vi "_PC_Daemon_Turbo stateMachine.vi"(5 "state":T1, 7 "engMode":bool, 8 "error in":errorcluster, 10 "newData":variant, 11 "refnumCluster":T2) -> (0 "error out":errorcluster)   [LabVIEW 2018]
uses:
  turboState.ctl
  RT/PublicSubVI/Ctl/_ctl_RT_TurboSettings.ctl
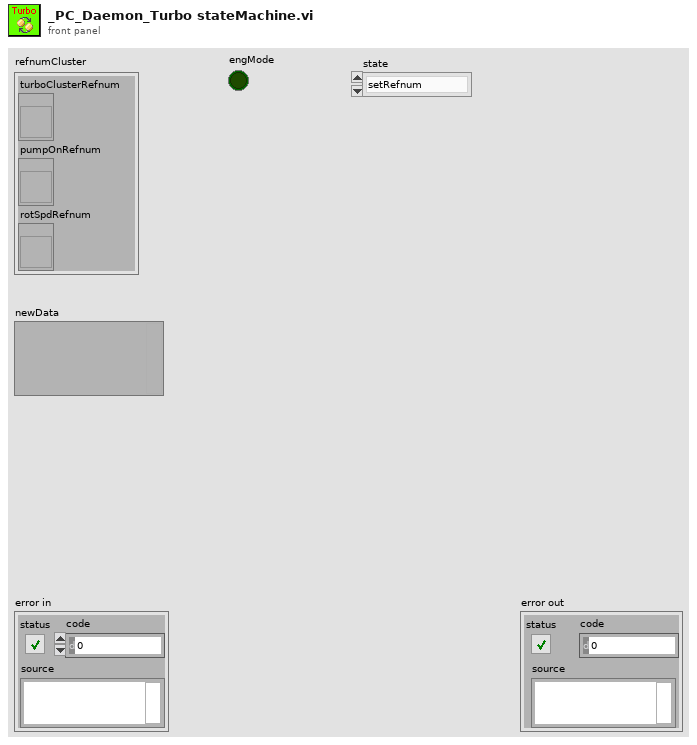
[diagram p1: front panel]
types:
  T1 = typedef "turboState.ctl" = enum16{"setRefnum", "init", "setParam", "close"}
  T2 = cluster{"turboClusterRefnum":refnum<vi>, "pumpOnRefnum":refnum<vi>, "rotSpdRefnum":refnum<vi>}
  T3 = typedef "_ctl_RT_TurboSettings.ctl" = cluster{"Preset rot. speed \nat standby mode(%)":dbl, "Speed set value in rot. speed \nsetting operations (%)":dbl, "Max. power (%)":dbl, "Gas mode: ":enum16{"heavy", "light", "helium"}, "Operations mode: ":bool, "Motor turbopump: ":bool, "Pumping station: ":bool, "Standby: ":bool, "Timestamp":timestamp}
  T4 = cluster{"Preset rot. speed \nat standby mode(%)":dbl, "Speed set value in rot. speed \nsetting operations (%)":dbl, "Max. power (%)":dbl, "Gas mode: ":enum16{"heavy", "light", "helium"}, "Operations mode: ":bool, "Motor turbopump: ":bool, "Pumping station: ":bool, "Standby: ":bool}
  T5 = enum8{"Enabled", "Disabled", "Disabled and Grayed Out"}
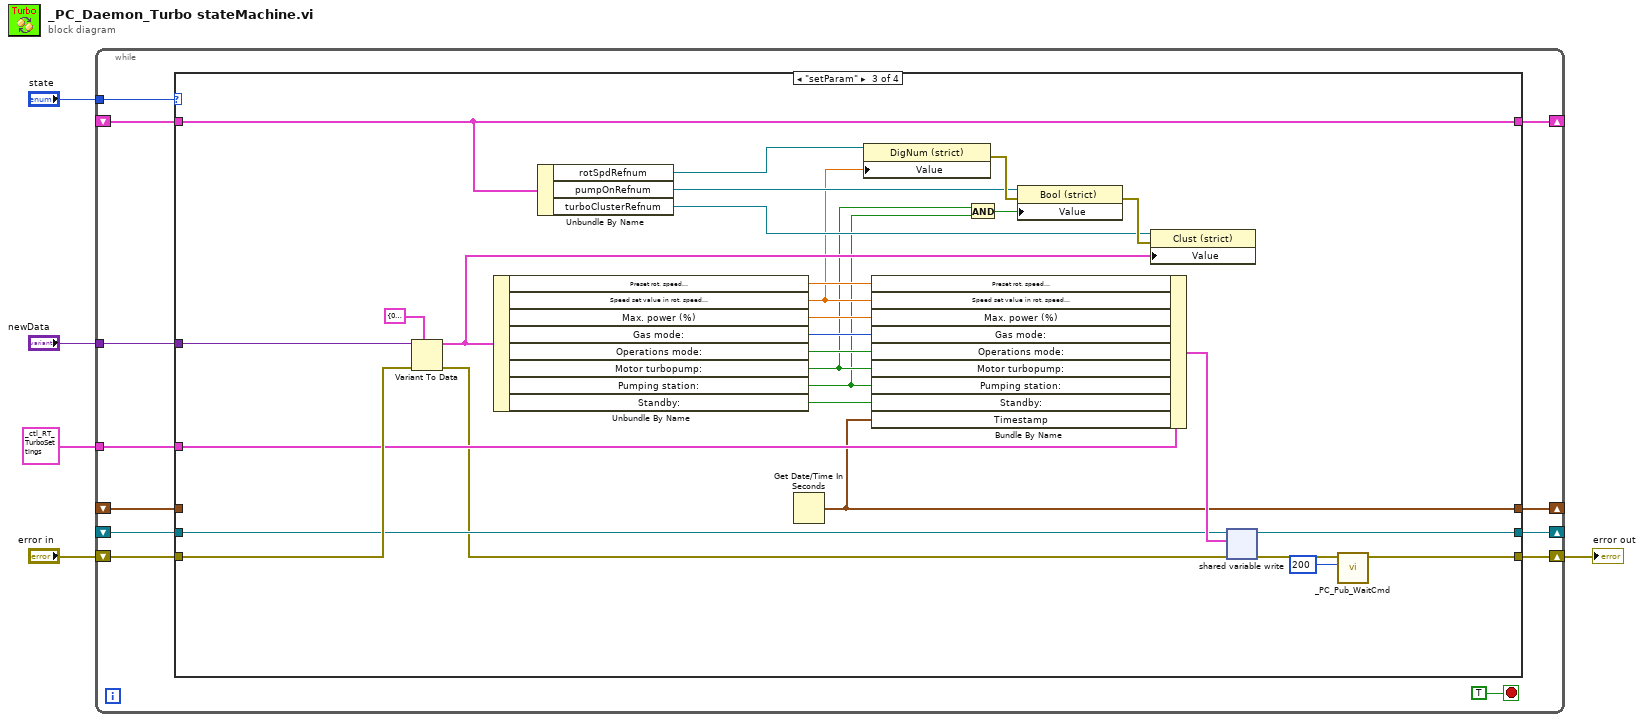
[diagram p0: block diagram]
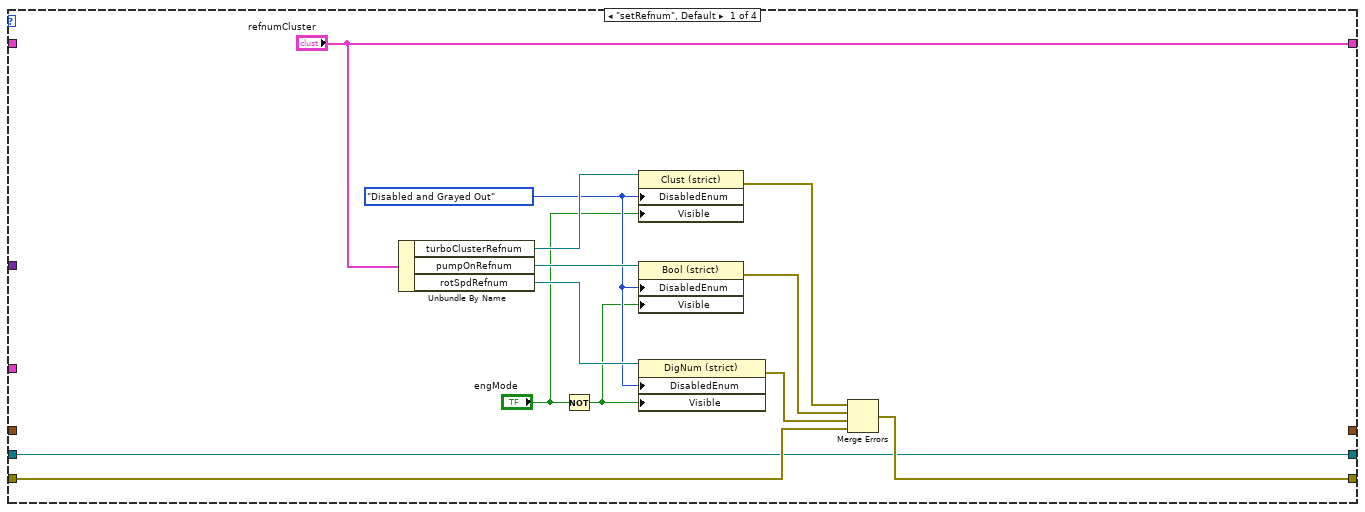
[diagram p2: hidden frame]
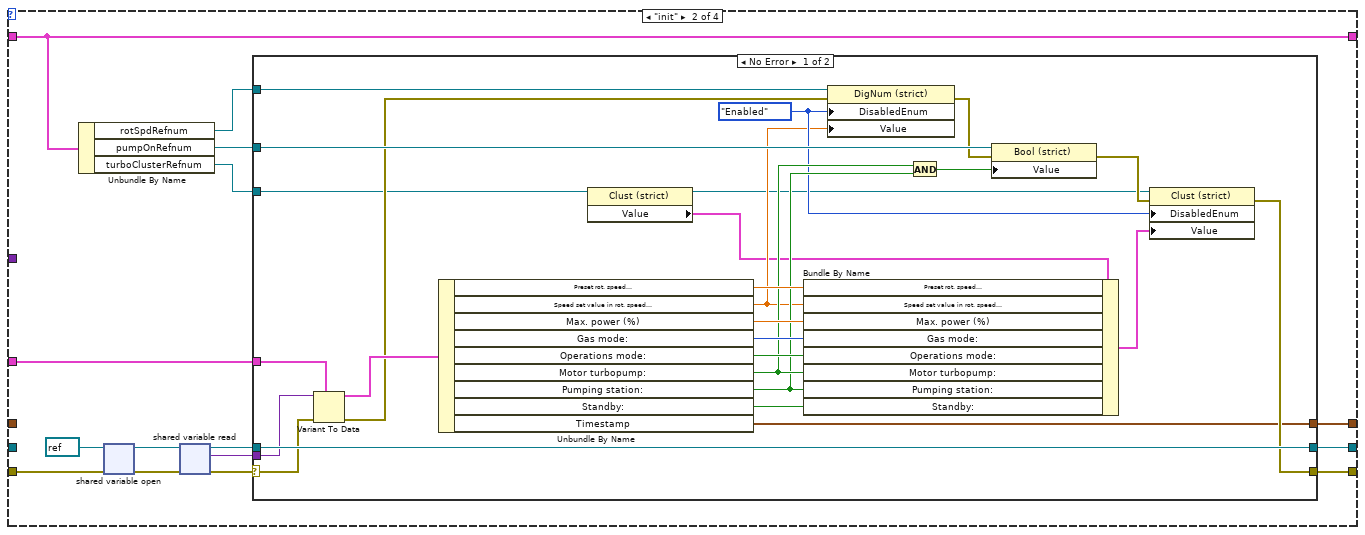
[diagram p3: hidden frame]
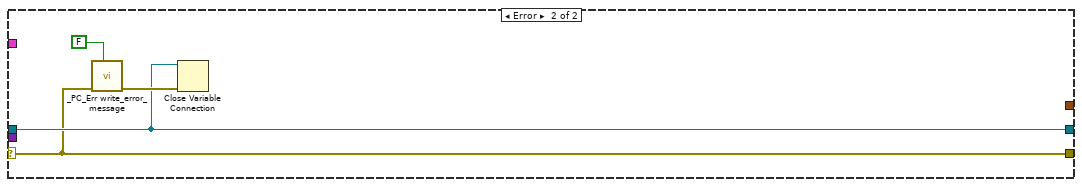
[diagram p4: hidden frame]
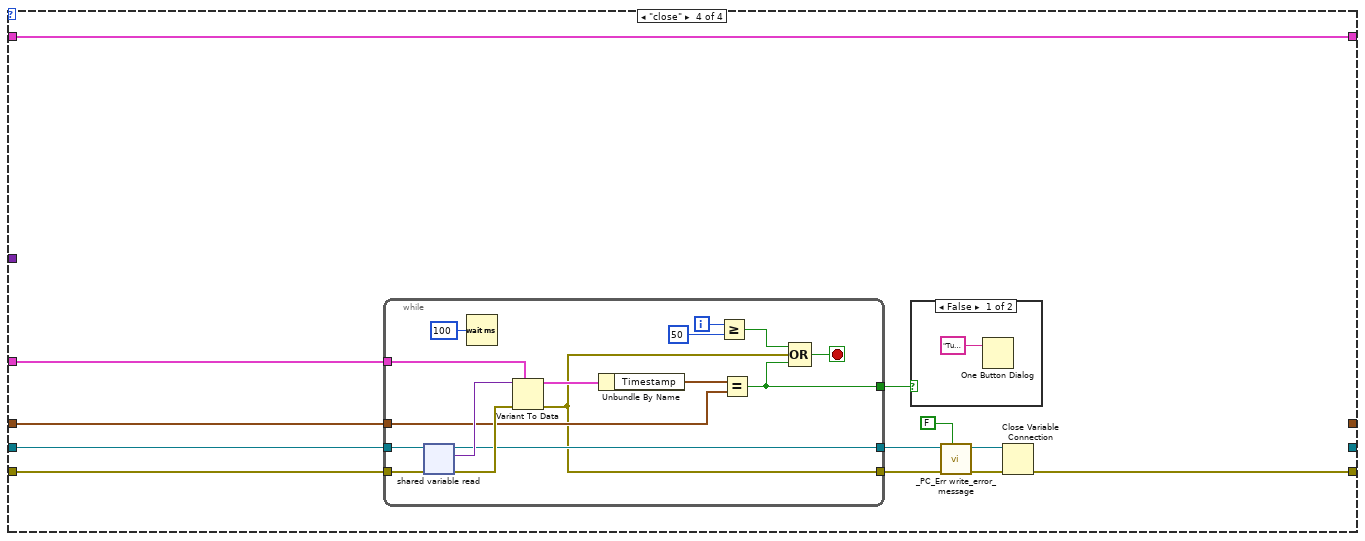
[diagram p5: hidden frame]
diagram:
  n1 = while {
    tunnel: "state" -> [w17]
    shift-right: [w16] -> _
    shift-left: _ -> [w13]
    shift-right: [w15] -> w2
    shift-left: "error in" -> [w14]
    tunnel: T3 {"Preset rot. speed \nat standby mode(%)"=0.0, "Speed set value in rot. speed \nsetting operations (%)"=0.0, "Max. power (%)"=0.0, "Gas mode: "=enum."heavy", "Operations mode: "=FALSE, "Motor turbopump: "=FALSE, "Pumping station: "=FALSE, "Standby: "=FALSE, "Timestamp"=timestamp(0 s since 1904-01-01)} ("TurboSettings") -> [w12]
    shift-right: [w11] -> _
    shift-left: _ -> [w10]
    tunnel: "newData" -> [w9]
    shift-right: [w7] -> _
    shift-left: _ -> [w6]
    stop <- TRUE stop-if-true
    n2 = case shown="\"setParam\"" w17 {
      tunnel: ["refnumCluster" w36 w87 w111] -> w16
      tunnel: [w20 w35 w77 w105] -> w15
      tunnel: w14 -> [w19 w32 w101 w113]
      tunnel: w13 -> [_ w36 w87 w111]
      tunnel: w12 -> [_ w40 w100 w110]
      tunnel: [w18 w34 w80 _] -> w11
      tunnel: w10 -> [w18 _ w82 w114]
      tunnel: w9 -> [_ _ w102 _]
      tunnel: [_ w31 w76 _] -> w7
      tunnel: w6 -> [_ _ _ w112]
      frame "setRefnum", Default {
        w26 = T5."Disabled and Grayed Out" ("Disabled")
        n3 = Unbundle By Name("refnumCluster") -> ("turboClusterRefnum"=w27:refnum<vi>, "pumpOnRefnum"=w28:refnum<vi>, "rotSpdRefnum"=w29:refnum<vi>)
        n4 = Not(x="engMode") -> (.not. x?=w25:bool)
        n5 = property class="Clust (strict)"(reference=w27, "DisabledEnum"=w26, "Visible"="engMode") -> (error out=w23:errorcluster)  [unwired: 1 in, 1 out]
        n6 = property class="Bool (strict)"(reference=w28, "DisabledEnum"=w26, "Visible"=w25) -> (error out=w22:errorcluster)  [unwired: 1 in, 1 out]
        n7 = property class="DigNum (strict)"(reference=w29, "DisabledEnum"=w26, "Visible"=w25) -> (error out=w21:errorcluster)  [unwired: 1 in, 1 out]
        n8 = Merge Errors(w23, w22, w21, w19) -> (w20:errorcluster)
      }
      frame "init" {
        n9 = Unbundle By Name(w36) -> ("rotSpdRefnum"=w37:refnum<vi>, "pumpOnRefnum"=w38:refnum<vi>, "turboClusterRefnum"=w39:refnum<vi>)
        n10 = shared-variable-open(refnum<k21> "ni.var.psp://NI-sbRIO/_RT_CtrlLoop_TurboPump_Variables/TurboSettings" ("shared variable refnum in"), w32) -> (w45:refnum<k21>, w44:errorcluster)
        n11 = shared-variable-read(w45, w44) -> (w43:refnum<k21>, w41:errorcluster, w42:variant)
        n12 = case shown="No Error" w41 {
          selector: w41 -> [w69 w72]
          tunnel: w43 -> [w71 w73]
          tunnel: [w71 w73] -> w34
          tunnel: w42 -> [w70 _]
          tunnel: w39 -> [w51 _]
          tunnel: w38 -> [w61 _]
          tunnel: w37 -> [w57 _]
          tunnel: w40 -> [w48 _]
          tunnel: [w47 w72] -> w35
          tunnel: [w46 _] -> w31
          frame No Error {
            w56 = T5."Enabled" ("Disabled")
            n13 = Variant To Data(error in=w69, type=w48, Variant=w70) -> (data=w68:T3, error out=w54:errorcluster)
            n14 = Unbundle By Name(w68) -> ("Preset rot. speed \nat standby mode(%)"=w67:dbl, "Speed set value in rot. speed \nsetting operations (%)"=w55:dbl, "Max. power (%)"=w66:dbl, "Gas mode:"=w65:enum16{"heavy", "light", "helium"}, "Operations mode:"=w64:bool, "Motor turbopump:"=w60:bool, "Pumping station:"=w59:bool, "Standby:"=w63:bool, "Timestamp"=w46:timestamp)
            n15 = property class="Clust (strict)"(reference=w51) -> (reference out=w50:refnum<vi>, "Value"=w49:T4)  [unwired: 1 in, 1 out]
            n16 = Bundle By Name(cluster=w49, "Preset rot. speed \nat standby mode(%)"=w67, "Speed set value in rot. speed \nsetting operations (%)"=w55, "Max. power (%)"=w66, "Gas mode:"=w65, "Operations mode:"=w64, "Motor turbopump:"=w60, "Pumping station:"=w59, "Standby:"=w63) -> (w62:T4)
            n17 = property class="DigNum (strict)"(reference=w57, error in=w54, "DisabledEnum"=w56, "Value"=w55) -> (error out=w53:errorcluster)  [unwired: 1 out]
            n18 = And(x=w60, y=w59) -> (x .and. y?=w58:bool)
            n19 = property class="Bool (strict)"(reference=w61, error in=w53, "Value"=w58) -> (error out=w52:errorcluster)  [unwired: 1 out]
            n20 = property class="Clust (strict)"(reference=w50, error in=w52, "DisabledEnum"=w56, "Value"=w62) -> (error out=w47:errorcluster)  [unwired: 1 out]
          }
          frame Error {
            n21 = call "_PC_Err write_error_message.vi"("show msg( T )"=FALSE, "error in"=w72) -> ("error out"=w75:errorcluster)  [unwired: 9 in]
            n22 = Close Variable Connection(8:w75, 11:w73) -> ()  [unwired: 1 out]
          }
        }
      }
      frame "setParam" {
        n23 = Variant To Data(error in=w101, type=T4 {"Preset rot. speed \nat standby mode(%)"=0.0, "Speed set value in rot. speed \nsetting operations (%)"=0.0, "Max. power (%)"=0.0, "Gas mode: "=enum."heavy", "Operations mode: "=FALSE, "Motor turbopump: "=FALSE, "Pumping station: "=FALSE, "Standby: "=FALSE} ("TC110 Settings"), Variant=w102) -> (data=w88:T4, error out=w81:errorcluster)
        n24 = Unbundle By Name(w88) -> ("Preset rot. speed \nat standby mode(%)"=w99:dbl, "Speed set value in rot. speed \nsetting operations (%)"=w86:dbl, "Max. power (%)"=w98:dbl, "Gas mode:"=w97:enum16{"heavy", "light", "helium"}, "Operations mode:"=w96:bool, "Motor turbopump:"=w85:bool, "Pumping station:"=w84:bool, "Standby:"=w95:bool)
        n25 = Unbundle By Name(w87) -> ("rotSpdRefnum"=w89:refnum<vi>, "pumpOnRefnum"=w90:refnum<vi>, "turboClusterRefnum"=w91:refnum<vi>)
        n26 = Get Date/Time In Seconds() -> (seconds since 1Jan1904=w76:timestamp)
        n27 = property class="DigNum (strict)"(reference=w89, "Value"=w86) -> (error out=w93:errorcluster)  [unwired: 1 in, 1 out]
        n28 = Bundle By Name(cluster=w100, "Preset rot. speed \nat standby mode(%)"=w99, "Speed set value in rot. speed \nsetting operations (%)"=w86, "Max. power (%)"=w98, "Gas mode:"=w97, "Operations mode:"=w96, "Motor turbopump:"=w85, "Pumping station:"=w84, "Standby:"=w95, "Timestamp"=w76) -> (w83:T3)
        n29 = And(x=w85, y=w84) -> (x .and. y?=w94:bool)
        n30 = property class="Bool (strict)"(reference=w90, error in=w93, "Value"=w94) -> (error out=w92:errorcluster)  [unwired: 1 out]
        n31 = property class="Clust (strict)"(reference=w91, error in=w92, "Value"=w88) -> ()  [unwired: 2 out]
        n32 = shared-variable-write(w82, w81, w83) -> (w80:refnum<k21>, w78:errorcluster)
        n33 = call "_PC_Pub_WaitCmd.vi"("milliseconds to wait"=u32 200, "error in (no error)"=w78) -> ("error out"=w77:errorcluster)  [unwired: 9 in]
      }
      frame "close" {
        n34 = while {
          tunnel: w114 -> [w131]
          tunnel: [w127] -> w107
          tunnel: w112 -> [w124]
          tunnel: w110 -> [w123]
          tunnel: w113 -> [w130]
          tunnel: [w118] -> w106
          tunnel: [w116] -> w104
          i -> [w122]
          stop <- w117 stop-if-true
          n35 = shared-variable-read(w131, w130) -> (w127:refnum<k21>, w128:errorcluster, w129:variant)
          n36 = Wait (ms)(milliseconds to wait=u32 100) -> ()  [unwired: 1 out]
          n37 = Variant To Data(error in=w128, type=w123, Variant=w129) -> (data=w126:T3, error out=w118:errorcluster)
          n38 = Unbundle By Name(w126) -> ("Timestamp"=w125:timestamp)
          n39 = Greater Or Equal?(x=w122, y=50) -> (x >= y?=w119:bool)
          n40 = Equal?(x=w125, y=w124) -> (x = y?=w116:bool)
          n41 = Compound Arithmetic op=OR(w119, w118, w116) -> (w117:bool)
        }
        n42 = case shown="False" w104 {
          frame False {
            n43 = One Button Dialog(message="Turbo setup is not complete") -> ()  [unwired: 1 in, 1 out]
          }
          frame True {
          }
        }
        n44 = call "_PC_Err write_error_message.vi"("show msg( T )"=FALSE, "error in"=w106) -> ("error out"=w109:errorcluster)  [unwired: 9 in]
        n45 = Close Variable Connection(8:w109, 11:w107) -> (0:w105:errorcluster)
      }
    }
  }
  "error out" <- w2
